vi "Get Config.vi"(8 "error in (no error)":errorcluster, 11 "AD4212C in":refnum<class "AD4212C.lvclass">) -> (0 "error out":errorcluster, 1 "Config Data":variant, 3 "AD4212C out":refnum<class "AD4212C.lvclass">)   [LabVIEW 2014, in "AD4212C.lvlib" / "AD4212C.lvclass"]
uses:
  AD4212C.lvclass
  AD4212C.lvclass/AD4212C.ctl
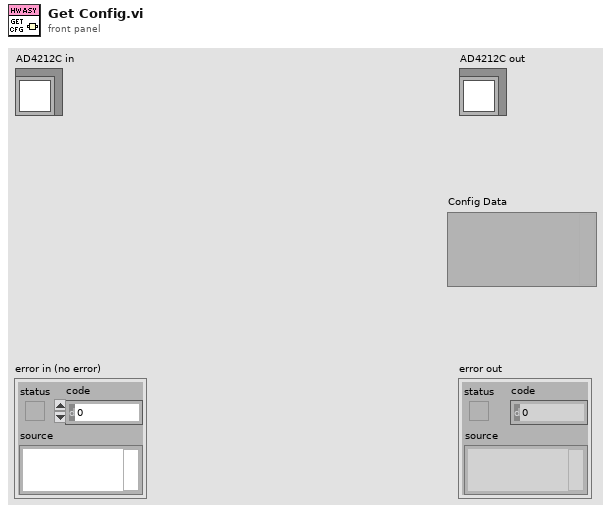
[diagram p1: front panel]
types:
  T1 = typedef "AD4212C Lib.lvlib/Connection Data.ctl" = cluster{"Conection Data":refnum<visa-resource-name>}
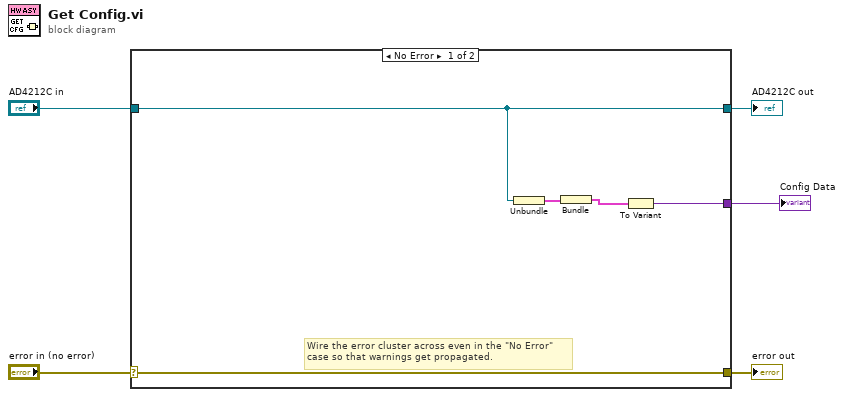
[diagram p0: block diagram]
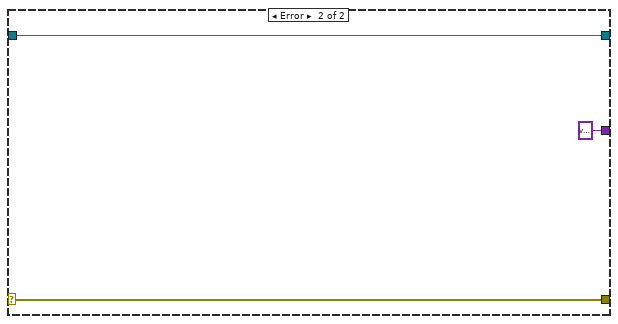
[diagram p2: hidden frame]
diagram:
  n1 = case shown="No Error" "error in (no error)" {
    selector: "error in (no error)" -> [w10 w13]
    tunnel: [w10 w13] -> w4
    tunnel: [w7 w12] -> w2
    tunnel: "AD4212C in" -> [w7 w12]
    tunnel: [w9 variant ("Variant")] -> w1
    frame No Error {
      # "Wire the error cluster across even in the \"No Error\"\ncase so that warnings get propagated."
      n2 = Unbundle(w7) -> (w8:T1)
      n3 = Bundle("Connection Data"=w8) -> (w6:cluster{"Connection Data":T1})  [unwired: 1 in]
      n4 = To Variant(anything=w6) -> (Variant=w9:variant)
    }
    frame Error {
    }
  }
  "error out" <- w4
  "AD4212C out" <- w2
  "Config Data" <- w1
